vi "Logging Control.vi"() -> ()   [LabVIEW 2016]
uses:
  <vilib>/Message/Open (Sync).vi
  <vilib>/Message/Unsubscribe (Sync).vi
  <vilib>/Message/Subscribe (Sync).vi
  <vilib>/TagLibrary/Write (String).vi
  <vilib>/TagLibrary/Write (Double).vi
  <vilib>/TagLibrary/Write (Int).vi
  <vilib>/Message/Publish (Sync).vi
  <vilib>/TagLibrary/Read Int Values.vi
  <vilib>/TagLibrary/Read String Values.vi
  <vilib>/TagLibrary/Read Double Values.vi
  <vilib>/TagLibrary/Tag Library.lvlib
panel:
  out "Buffer":i32
  in  "Log":bool
  in  "Sample Rate":dbl=1000.0 format="%0.2f"
  in  "Channel":string(combo)
  in  "Refresh":bool
  in  "System":string(combo)
  in  "Close":bool
  out "Status":string
  out "Files Sent":i32
  in  "Send File":bool
  in  "Start":bool
  out "Iteration":i32
  out "Waveform Graph":waveform(dbl)(graph)
  in  "Stop":bool
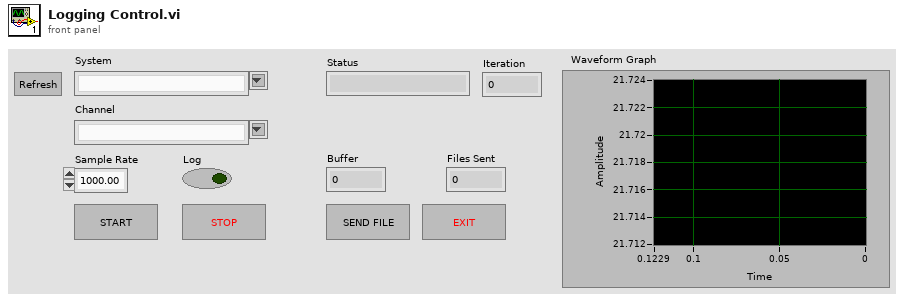
[diagram p1: front panel]
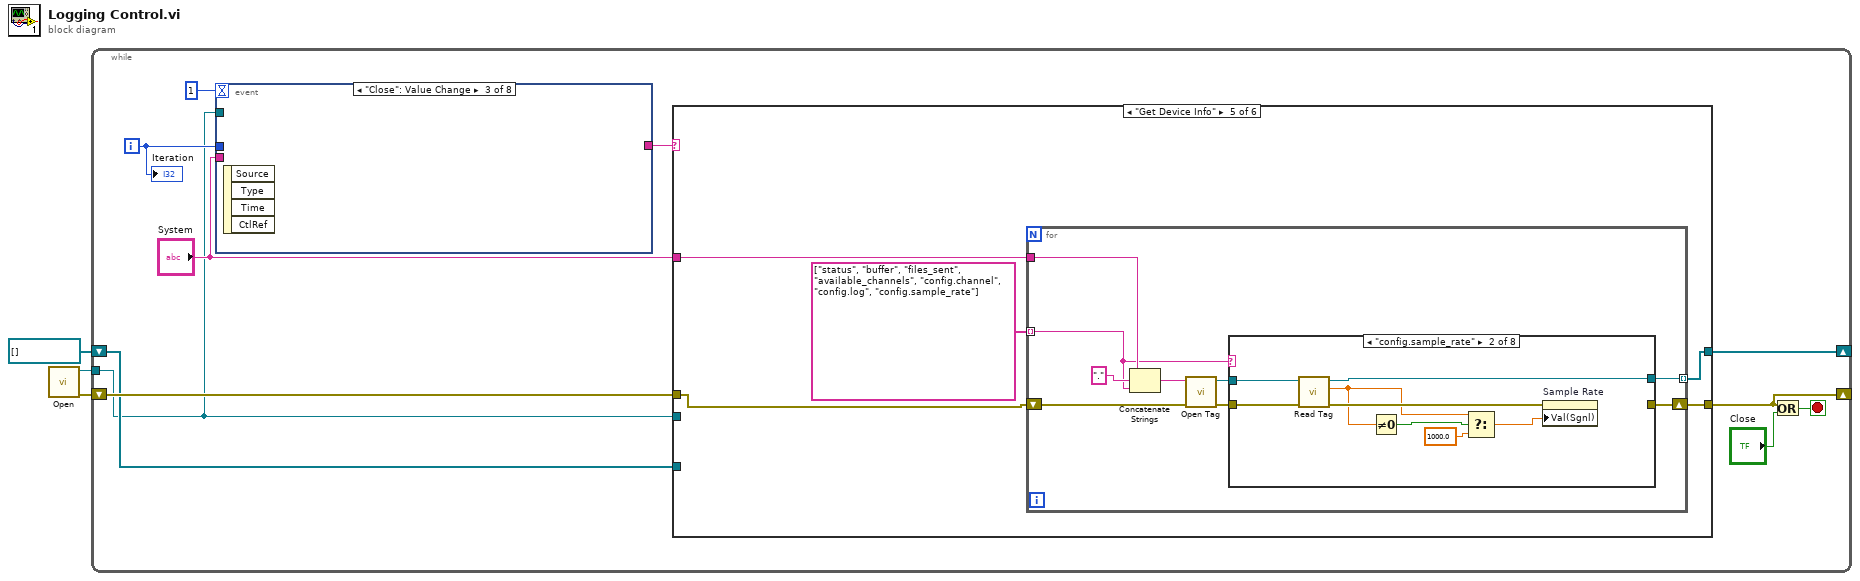
[diagram p0: block diagram]
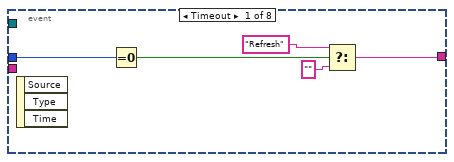
[diagram p2: hidden frame]
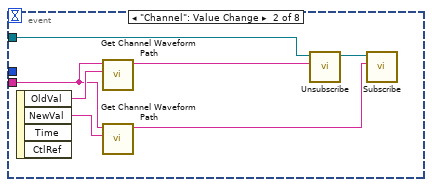
[diagram p3: hidden frame]
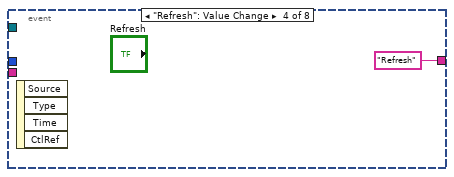
[diagram p4: hidden frame]
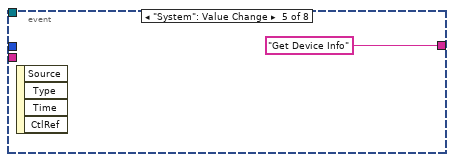
[diagram p5: hidden frame]
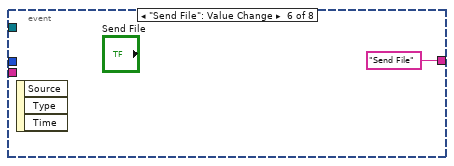
[diagram p6: hidden frame]
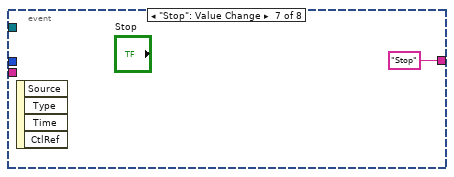
[diagram p7: hidden frame]
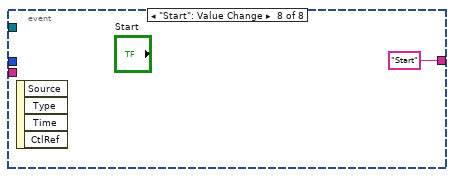
[diagram p8: hidden frame]
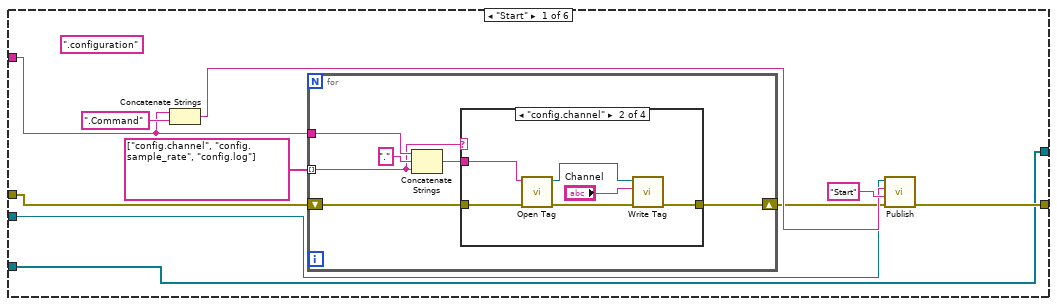
[diagram p9: hidden frame]
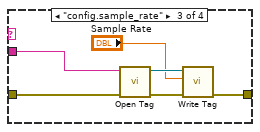
[diagram p11: hidden frame]
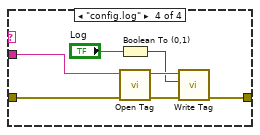
[diagram p12: hidden frame]
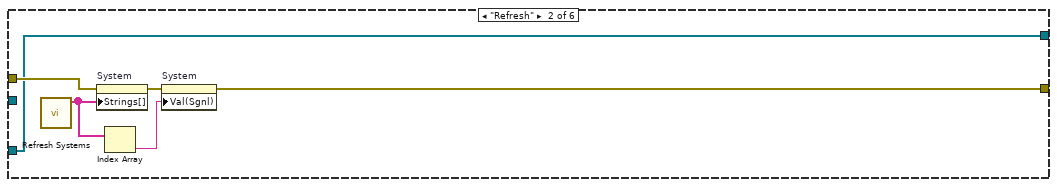
[diagram p13: hidden frame]
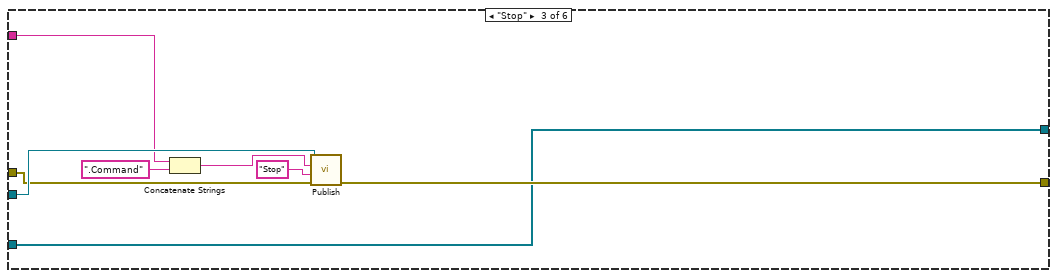
[diagram p14: hidden frame]
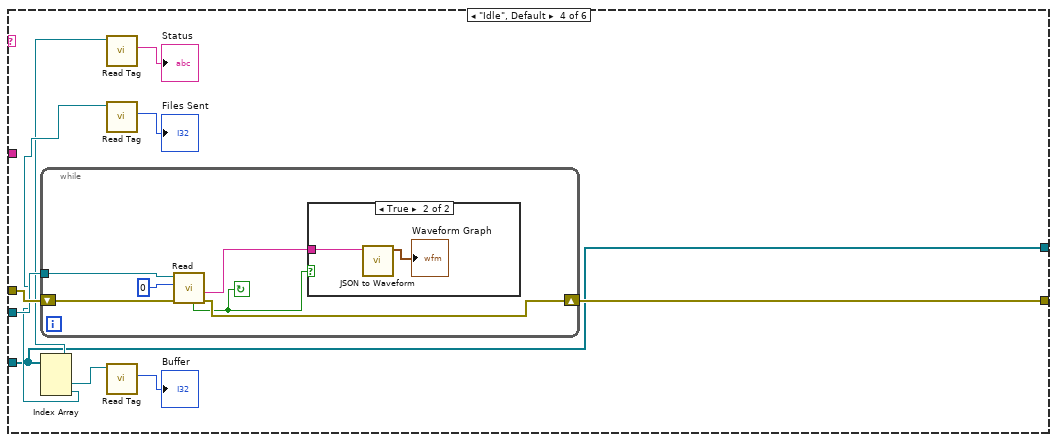
[diagram p15: hidden frame]
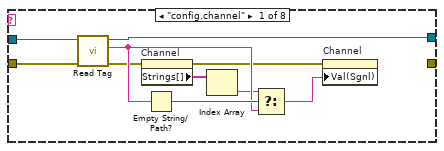
[diagram p17: hidden frame]
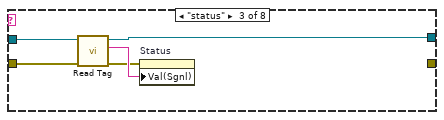
[diagram p18: hidden frame]
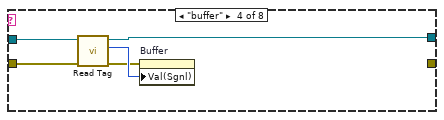
[diagram p19: hidden frame]
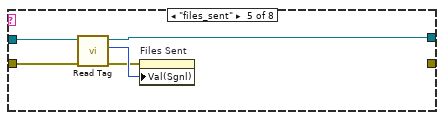
[diagram p20: hidden frame]
diagram:
  n1 = call-poly <vilib>:"Open.vi"() -> ("error out"=w2:errorcluster, "Message Sync Refnum"=w3:refnum<k21>)  [unwired: 10 in]
  n2 = while {
    shift-right: [w9] -> _
    shift-left: w2 -> [w14]
    tunnel: w3 -> [w4]
    shift-right: [w6] -> _
    shift-left: refnum<k21>[] [] -> [w7]
    i -> [w11]
    stop <- w10 stop-if-true
    n3 = event shown="[2] \"Close\": Value Change" {
      selector: _ -> [_ _ _ _ _ _ _ _]
      dyn-events: _ -> [_ _ _ _ _ _ _ _]
      timeout: 1 -> [_ _ _ _ _ _ _ _]
      tunnel: [w15 _ _ "Refresh" ("topic") "Get Device Info" ("topic") "Send File" ("topic") "Stop" ("topic") "Start" ("topic")] -> w12
      tunnel: w11 -> [w18 _ _ _ _ _ _ _]
      tunnel: "System" -> [_ w25 _ _ _ _ _ _]
      tunnel: w4 -> [_ w23 _ _ _ _ _ _]
      event Timeout {
        n4 = event-data() -> ()  [unwired: 1 in, 3 out]
        n5 = Equal To 0?(x=w18) -> (x = 0?=w19:bool)
        n6 = Select(t="Refresh", s=w19, f="") -> (s? t:f=w15:string)
      }
      event "Channel": Value Change {
        n7 = event-data() -> ("OldVal"=w26:string, "NewVal"=w24:string)  [unwired: 1 in, 2 out]
        n8 = call "Get Channel Waveform Path.vi"("Target"=w25, "Channel"=w26) -> ("Topic"=w21:string)  [unwired: 8 in]
        n9 = call "Get Channel Waveform Path.vi"("Target"=w25, "Channel"=w24) -> ("Topic"=w20:string)  [unwired: 8 in]
        n10 = call-poly <vilib>:"Unsubscribe.vi"("topic"=w21, "Message Sync Refnum"=w23) -> ("Message Sync Refnum"=w22:refnum<k21>)  [unwired: 8 in, 1 out]
        n11 = call-poly <vilib>:"Subscribe.vi"("topic"=w20, "Message Sync Refnum"=w22) -> ()  [unwired: 8 in, 2 out]
      }
      event "Close": Value Change {
        n12 = event-data() -> ()  [unwired: 1 in, 4 out]
      }
      event "Refresh": Value Change {
        n13 = event-data() -> ()  [unwired: 1 in, 4 out]
      }
      event "System": Value Change {
        n14 = event-data() -> ()  [unwired: 1 in, 4 out]
      }
      event "Send File": Value Change {
        n15 = event-data() -> ()  [unwired: 1 in, 3 out]
      }
      event "Stop": Value Change {
        n16 = event-data() -> ()  [unwired: 1 in, 4 out]
      }
      event "Start": Value Change {
        n17 = event-data() -> ()  [unwired: 1 in, 4 out]
      }
    }
    n18 = case shown="\"Get Device Info\"" w12 {
      tunnel: w14 -> [w33 w73 w79 w90 w103 w169]
      tunnel: [w41 w71 w80 w91 w101 w170] -> w9
      tunnel: w4 -> [w36 _ w81 w89 _ w171]
      tunnel: "System" -> [w35 _ w77 _ w102 w166]
      tunnel: w7 -> [w40 w68 w78 w82 _ w168]
      tunnel: [w40 w68 w78 w82 w100 w168] -> w6
      frame "Start" {
        (unwired) ".configuration" ("string")
        n19 = Concatenate Strings(w35, ".Command" ("topic")) -> (w37:string)
        n20 = for {
          tunnel: w35 -> [w47]
          tunnel: string[] ["config.channel", "config.sample_rate", "config.log"] -> [w45] mode=indexing
          shift-right: [w42] -> w32
          shift-left: w33 -> [w43]
          n21 = Concatenate Strings(w47, "." ("string"), w45) -> (w44:string)
          n22 = case shown="\"config.channel\"" w45 {
            tunnel: w44 -> [_ w52 w58 w65]
            tunnel: w43 -> [w48 w50 w55 w62]
            tunnel: [w48 w49 w56 w61] -> w42
            frame "False", Default {
            }
            frame "config.channel" {
              n23 = call <vilib>:"Open Tag.vi"("error in (no error)"=w50, "tag path"=w52) -> ("error out"=w54:errorcluster, "tag reference out"=w53:refnum<k21>)  [unwired: 8 in]
              n24 = call-poly <vilib>:"Write Tag.vi"("error in (no error)"=w54, "string"="Channel", "tag reference in"=w53) -> ("error out"=w49:errorcluster)  [unwired: 7 in, 1 out]
            }
            frame "config.sample_rate" {
              n25 = call <vilib>:"Open Tag.vi"("error in (no error)"=w55, "tag path"=w58) -> ("error out"=w60:errorcluster, "tag reference out"=w59:refnum<k21>)  [unwired: 8 in]
              n26 = call-poly <vilib>:"Write Tag.vi"("error in (no error)"=w60, "double"="Sample Rate", "tag reference in"=w59) -> ("error out"=w56:errorcluster)  [unwired: 7 in, 1 out]
            }
            frame "config.log" {
              n27 = Boolean To (0,1)(Boolean="Log") -> (0, 1=w63:i16)
              n28 = call <vilib>:"Open Tag.vi"("error in (no error)"=w62, "tag path"=w65) -> ("error out"=w67:errorcluster, "tag reference out"=w66:refnum<k21>)  [unwired: 8 in]
              n29 = call-poly <vilib>:"Write Tag.vi"("error in (no error)"=w67, "int"=w63, "tag reference in"=w66) -> ("error out"=w61:errorcluster)  [unwired: 7 in, 1 out]
            }
          }
        }
        n30 = call-poly <vilib>:"Publish.vi"("error in (no error)"=w32, "message"="Start" ("topic"), "topic"=w37, "Message Sync Refnum"=w36) -> ("error out"=w41:errorcluster)  [unwired: 6 in, 1 out]
      }
      frame "Refresh" {
        n31 = call "Refresh Systems.vi"() -> ("Systems"=w70:string[])  [unwired: 11 in]
        n32 = property on="System" class="CmbBox"(error in=w73, "Strings[]"=w70) -> (error out=w72:errorcluster)  [unwired: 1 in, 1 out]
        n33 = Index Array(array=w70) -> (element=w69:string)  [unwired: 1 in]
        n34 = property on="System" class="CmbBox"(error in=w72, "Val(Sgnl)"=w69) -> (error out=w71:errorcluster)  [unwired: 1 in, 1 out]
      }
      frame "Stop" {
        n35 = Concatenate Strings(w77, ".Command" ("topic")) -> (w74:string)
        n36 = call-poly <vilib>:"Publish.vi"("error in (no error)"=w79, "message"="Stop" ("topic"), "topic"=w74, "Message Sync Refnum"=w81) -> ("error out"=w80:errorcluster)  [unwired: 6 in, 1 out]
      }
      frame "Idle", Default {
        n37 = while {
          tunnel: w89 -> [w95]
          shift-right: [w97] -> w91
          shift-left: w90 -> [w96]
          stop <- w92 continue-if-true
          n38 = call <vilib>:"Read.vi"("error in (no error)"=w96, "timeoutMilliseconds"=0, "Message Sync Refnum"=w95) -> ("error out"=w97:errorcluster, "message"=w94:string, "dequeueStatus"=w92:bool)  [unwired: 4 in, 2 out]
          n39 = case shown="True" w92 {
            tunnel: w94 -> [_ w99]
            frame False {
            }
            frame True {
              n40 = call "JSON to Waveform.vi"("message"=w99) -> ("Waveform"=→"Waveform Graph":waveform(dbl))  [unwired: 10 in]
            }
          }
        }
        n41 = Index Array(array=w82) -> (element #1=w83:refnum<k21>, element #2=w84:refnum<k21>, element #3=w85:refnum<k21>)  [unwired: 3 in]
        n42 = call-poly <vilib>:"Read Tag.vi"("tag reference in"=w83) -> ("string"=→"Status":string)  [unwired: 7 in, 3 out]
        n43 = call-poly <vilib>:"Read Tag.vi"("tag reference in"=w85) -> ("integer"=→"Files Sent":i32)  [unwired: 6 in, 4 out]
        n44 = call-poly <vilib>:"Read Tag.vi"("tag reference in"=w84) -> ("integer"=→"Buffer":i32)  [unwired: 6 in, 4 out]
      }
      frame "Get Device Info" {
        n45 = for {
          tunnel: w102 -> [w113]
          tunnel: string[] ["status", "buffer", "files_sent", "available_channels", "config.channel", "config.log", "config.sample_rate"] -> [w108] mode=indexing
          shift-right: [w107] -> w101
          shift-left: w103 -> [w111]
          tunnel: [w105] -> w100 mode=indexing
          n46 = Concatenate Strings(w113, "." ("string"), w108) -> (w109:string)
          n47 = call <vilib>:"Open Tag.vi"("error in (no error)"=w111, "tag path"=w109) -> ("error out"=w110:errorcluster, "tag reference out"=w106:refnum<k21>)  [unwired: 8 in]
          n48 = case shown="\"config.sample_rate\"" w108 {
            tunnel: w110 -> [w122 w129 w133 w138 w143 w151 w155 w157]
            tunnel: [_ _ _ _ _ _ w155 _] -> w107
            tunnel: w106 -> [w123 w131 w136 w141 w146 w153 w154 w158]
            tunnel: [w121 w128 w132 w137 w142 w147 w154 w156] -> w105
            frame "config.channel" {
              n49 = call-poly <vilib>:"Read Tag.vi"("error in (no error)"=w122, "tag reference in"=w123) -> ("error out"=w115:errorcluster, "string"=w118:string, "tag reference out"=w121:refnum<k21>)  [unwired: 6 in, 1 out]
              n50 = property on="Channel" class="CmbBox"(error in=w115) -> (error out=w114:errorcluster, "Strings[]"=w117:string[])  [unwired: 1 in, 1 out]
              n51 = Empty String/Path?(string/path=w118) -> (empty?=w120:bool)
              n52 = Index Array(array=w117) -> (element=w116:string)  [unwired: 1 in]
              n53 = Select(t=w116, s=w120, f=w118) -> (s? t:f=w119:string)
              n54 = property on="Channel" class="CmbBox"(error in=w114, "Val(Sgnl)"=w119) -> ()  [unwired: 1 in, 2 out]
            }
            frame "config.sample_rate" {
              n55 = call-poly <vilib>:"Read Tag.vi"("error in (no error)"=w129, "tag reference in"=w131) -> ("error out"=w130:errorcluster, "double"=w126:dbl, "tag reference out"=w128:refnum<k21>)  [unwired: 5 in, 2 out]
              n56 = Not Equal To 0?(x=w126) -> (x != 0?=w127:bool)
              n57 = Select(t=w126, s=w127, f=1000.0) -> (s? t:f=w124:dbl)
              n58 = property on="Sample Rate" class="DigNum (strict)"(error in=w130, "Val(Sgnl)"=w124) -> ()  [unwired: 1 in, 2 out]
            }
            frame "status" {
              n59 = call-poly <vilib>:"Read Tag.vi"("error in (no error)"=w133, "tag reference in"=w136) -> ("error out"=w134:errorcluster, "string"=w135:string, "tag reference out"=w132:refnum<k21>)  [unwired: 6 in, 1 out]
              n60 = property on="Status" class="Str"(error in=w134, "Val(Sgnl)"=w135) -> ()  [unwired: 1 in, 2 out]
            }
            frame "buffer" {
              n61 = call-poly <vilib>:"Read Tag.vi"("error in (no error)"=w138, "tag reference in"=w141) -> ("error out"=w139:errorcluster, "integer"=w140:i32, "tag reference out"=w137:refnum<k21>)  [unwired: 5 in, 2 out]
              n62 = property on="Buffer" class="DigNum (strict)"(error in=w139, "Val(Sgnl)"=w140) -> ()  [unwired: 1 in, 2 out]
            }
            frame "files_sent" {
              n63 = call-poly <vilib>:"Read Tag.vi"("error in (no error)"=w143, "tag reference in"=w146) -> ("error out"=w144:errorcluster, "integer"=w145:i32, "tag reference out"=w142:refnum<k21>)  [unwired: 5 in, 2 out]
              n64 = property on="Files Sent" class="DigNum (strict)"(error in=w144, "Val(Sgnl)"=w145) -> ()  [unwired: 1 in, 2 out]
            }
            frame "config.log" {
              n65 = call-poly <vilib>:"Read Tag.vi"("error in (no error)"=w151, "tag reference in"=w153) -> ("error out"=w152:errorcluster, "integer"=w150:i32, "tag reference out"=w147:refnum<k21>)  [unwired: 5 in, 2 out]
              n66 = Number To Boolean Array(number=w150) -> (Boolean array=w149:bool[])
              n67 = Index Array(array=w149) -> (element=w148:bool)  [unwired: 1 in]
              n68 = property on="Log" class="Bool (strict)"(error in=w152, "Val(Sgnl)"=w148) -> ()  [unwired: 1 in, 2 out]
            }
            frame Default {
            }
            frame "available_channels" {
              n69 = call-poly <vilib>:"Read Tag.vi"("error in (no error)"=w157, "tag reference in"=w158) -> ("error out"=w160:errorcluster, "string"=w161:string, "tag reference out"=w156:refnum<k21>)  [unwired: 6 in, 1 out]
              n70 = Unflatten From JSON(JSON string=w161, type and defaults=string[] [], error in (no error)=w160) -> (value=w162:string[], error out=w159:errorcluster)  [unwired: 4 in]
              n71 = property on="Channel" class="CmbBox"(error in=w159, "Strings[]"=w162) -> ()  [unwired: 1 in, 2 out]
            }
          }
        }
      }
      frame "Send File" {
        n72 = Concatenate Strings(w166, ".Command" ("topic")) -> (w164:string)
        n73 = call-poly <vilib>:"Publish.vi"("error in (no error)"=w169, "message"="Send File" ("topic"), "topic"=w164, "Message Sync Refnum"=w171) -> ("error out"=w170:errorcluster)  [unwired: 6 in, 1 out]
      }
    }
    n74 = Or(x=w9, y="Close") -> (x .or. y?=w10:bool)
    "Iteration" <- w11
  }
